vi "05.1-3 INI Files with Multiple Keys.vi"() -> ()   [LabVIEW 2019]
uses:
  <vilib>/Utility/config.llb/Write Key (String).vi
  <vilib>/Utility/config.llb/Write Key (Double).vi
  <vilib>/Utility/config.llb/Write Key (I32).vi
  <vilib>/Utility/config.llb/NI_LVConfig.lvlib
panel:
  out "Config File Out":path
  in  "AO Channel":string
  in  "Samples per Channel":i32
  in  "Sample Rate":dbl
  in  "AI Channel":string
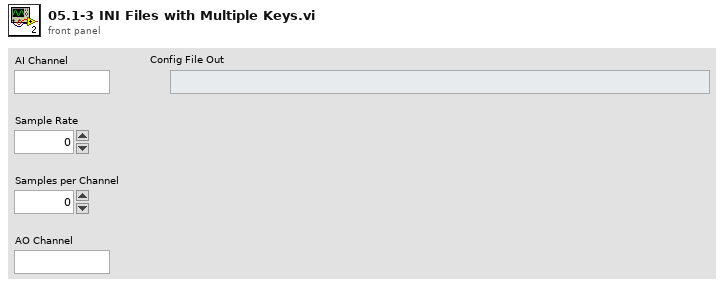
[diagram p1: front panel]
types:
  T1 = typedef "NI_LVConfig.lvlib/Config Data RefNum.ctl" = refnum<k1>
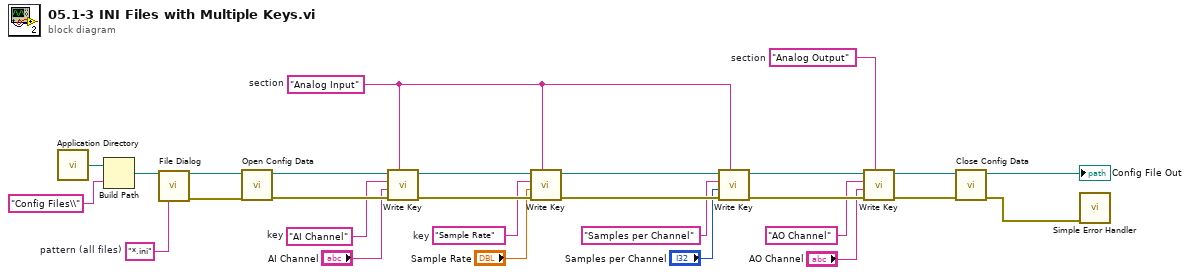
[diagram p0: block diagram]
diagram:
  w10 = "Analog Output"  # section
  w17 = "Sample Rate"  # key
  w13 = "Analog Input"  # section
  w21 = "AI Channel"  # key
  w28 = "*.ini"  # pattern (all files)
  n1 = call <vilib>:"Application Directory.vi"() -> ("Application Directory"=w27:path)
  n2 = Build Path(base path=w27, name or relative path="Config Files\\") -> (appended path=w1:path)
  n3 = call "File Dialog"("start path"=w1, "pattern (all files)"=w28) -> ("selected path"=w25:path, "error out"=w24:errorcluster)  [unwired: 10 in, 2 out]
  n4 = call <vilib>:"Open Config Data.vi"("error in (no error)"=w24, "configuration file path"=w25) -> ("error out"=w22:errorcluster, "refnum"=w23:T1)  [unwired: 7 in, 1 out]
  n5 = call-poly <vilib>:"Write Key.vi"("section"=w13, "error in (no error)"=w22, "value"="AI Channel", "key"=w21, "refnum"=w23) -> ("error out"=w19:errorcluster, "refnum out"=w18:T1)  [unwired: 4 in, 1 out]
  n6 = call-poly <vilib>:"Write Key.vi"("section"=w13, "error in (no error)"=w19, "value"="Sample Rate", "key"=w17, "refnum"=w18) -> ("error out"=w15:errorcluster, "refnum out"=w14:T1)  [unwired: 4 in, 1 out]
  n7 = call-poly <vilib>:"Write Key.vi"("section"=w13, "error in (no error)"=w15, "value"="Samples per Channel", "key"="Samples per Channel", "refnum"=w14) -> ("error out"=w9:errorcluster, "refnum out"=w8:T1)  [unwired: 4 in, 1 out]
  n8 = call-poly <vilib>:"Write Key.vi"("section"=w10, "error in (no error)"=w9, "value"="AO Channel", "key"="AO Channel", "refnum"=w8) -> ("error out"=w5:errorcluster, "refnum out"=w4:T1)  [unwired: 4 in, 1 out]
  n9 = call <vilib>:"Close Config Data.vi"("error in (no error)"=w5, "refnum"=w4) -> ("error out"=w3:errorcluster, "file path"=→"Config File Out":path)  [unwired: 8 in]
  n10 = call <vilib>:"Simple Error Handler.vi"("error in (no error)"=w3) -> ()  [unwired: 4 in, 5 out]
